vi "Get Endpoints from Switches JSON.vi"(8 "error in":errorcluster, 10 "topology":string, 11 "switches json":string) -> (0 "error out":errorcluster, 3 "endpoints":string[](array[string]))   [LabVIEW 2020, in "SLSC Switch Scripting.lvlib"]
uses:
  SLSC Switch Scripting.lvlib
  <vilib>/SLSC_Switch/Initialize with Topology (Simulate).vi
  <vilib>/SLSC_Switch/SLSC Switch.lvlib
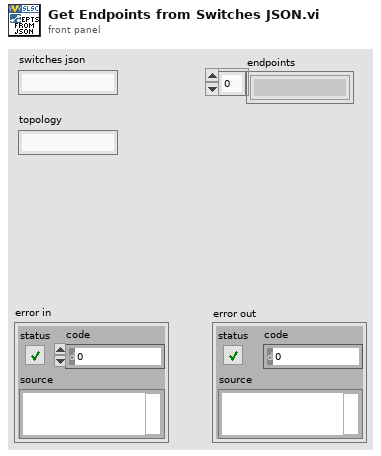
[diagram p1: front panel]
types:
  T1 = typedef "nislscslSession.ctl" = refnum<k20>
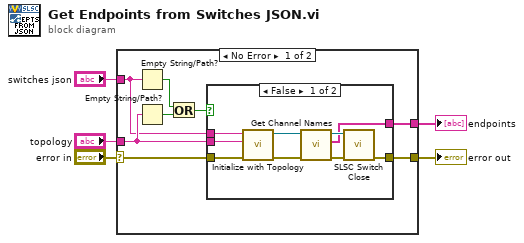
[diagram p0: block diagram]
diagram:
  n1 = case shown="No Error" "error in" {
    selector: "error in" -> [w13 w24]
    tunnel: "switches json" -> [w9 _]
    tunnel: "topology" -> [w10 _]
    tunnel: [w12 _] -> w2
    tunnel: [w11 w24] -> w1
    frame No Error {
      n2 = Empty String/Path?(string/path=w9) -> (empty?=w8:bool)
      n3 = Empty String/Path?(string/path=w10) -> (empty?=w7:bool)
      n4 = Or(x=w8, y=w7) -> (x .or. y?=w6:bool)
      n5 = case shown="False" w6 {
        tunnel: w13 -> [w22 w23]
        tunnel: [w17 _] -> w12
        tunnel: [w16 w23] -> w11
        tunnel: w10 -> [w15 _]
        tunnel: w9 -> [w14 _]
        frame False {
          n6 = call-poly <vilib>:"Initialize with Topology.vi"("error in (no error)"=w22, "topology"=w15, "switches json"=w14) -> ("error out"=w20:errorcluster, "session out"=w21:T1)  [unwired: 7 in]
          n7 = call <vilib>:"Get Channel Names.vi"("error in (no error)"=w20, "session in"=w21) -> ("error out"=w18:errorcluster, "channel names"=w17:string[], "session out"=w19:T1)  [unwired: 7 in]
          n8 = call "SLSC Switch Close.vi"("error in"=w18, "slsc switch session"=w19) -> ("error out"=w16:errorcluster)  [unwired: 9 in]
        }
        frame True {
        }
      }
    }
    frame Error {
    }
  }
  "error out" <- w1
  "endpoints" <- w2
